vi "Get Current Date.vi"() -> (1 "Day":string, 2 "Month":string, 3 "Year":string, 4 "Formatted Current Date":string)   [LabVIEW 2020]
panel:
  out "date string":string
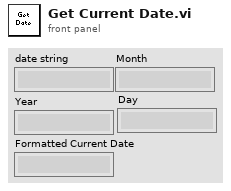
[diagram p1: front panel]
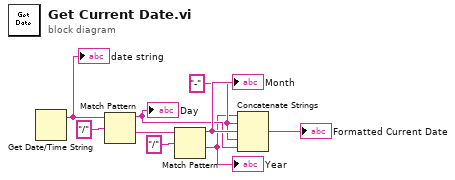
[diagram p0: block diagram]
diagram:
  w4 = "-" ("string")
  n1 = Get Date/Time String() -> (date string=w9:string)  [unwired: 3 in, 1 out]
  "date string" <- w9
  n2 = Match Pattern(string=w9, regular expression="/") -> (before substring=w2:string, after substring=w6:string)  [unwired: 1 in, 2 out]
  "Day" <- w2
  n3 = Match Pattern(string=w6, regular expression="/") -> (before substring=w5:string, after substring=w1:string)  [unwired: 1 in, 2 out]
  "Year" <- w1
  "Month" <- w5
  n4 = Concatenate Strings(w1, w4, w5, w4, w2) -> (→"Formatted Current Date":string)
